vi "Read DelayB.vi"(8 "error in (no error)":errorcluster, 11 "Trigger in":refnum<class "Trigger.lvclass">) -> (0 "error out":errorcluster, 2 "DelayB":string, 3 "Trigger out":refnum<class "Trigger.lvclass">)   [LabVIEW 2012, in "Trigger.lvclass"]
uses:
  Trigger.lvclass
  Trigger.lvclass/Trigger.ctl
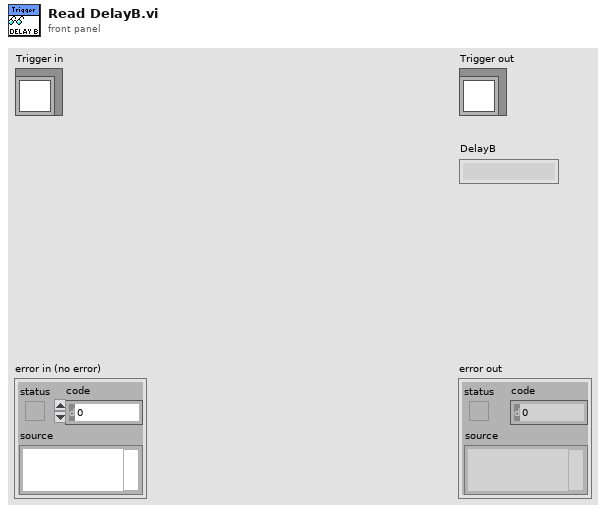
[diagram p1: front panel]
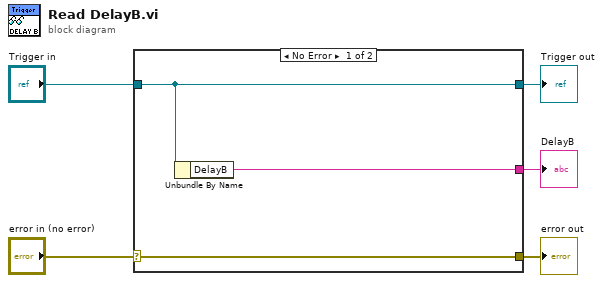
[diagram p0: block diagram]
diagram:
  n1 = case shown="No Error" "error in (no error)" {
    selector: "error in (no error)" -> [w8 w9]
    tunnel: [w8 w9] -> w4
    tunnel: [w7 w10] -> w2
    tunnel: "Trigger in" -> [w7 w10]
    tunnel: [w6 _] -> w1
    frame No Error {
      n2 = Unbundle By Name(w7) -> ("DelayB"=w6:string)
    }
    frame Error {
    }
  }
  "error out" <- w4
  "Trigger out" <- w2
  "DelayB" <- w1
